vi "Kill All Notifiers.vi"() -> ()   [LabVIEW 2019]
uses:
  Globals and TypeDefs/Type Definitions.llb/McPherson Status.ctt
  Globals and TypeDefs/Type Definitions.llb/3 way Status.ctl
panel:
  in  "Spectrometer Pos":T2
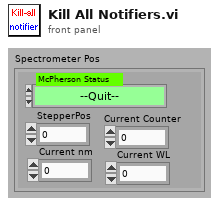
[diagram p1: front panel]
types:
  T1 = typedef "McPherson Status.ctt" = enum8{"--Quit--", "Error", "Initialization", "Standby", "Start Slew", "-Slew", "+Slew", "Slew Done", "Start Scan", "-Slew to Start", "+Slew to Start", "Scanning", "Scan Done", "Scan Pause", "Slew Pause", "Cancel", "Update Z0", "Sleep"}
  T2 = cluster{"StepperPos":i32, "Current nm":dbl, "Current Counter":dbl, "Current WL":dbl, "McPherson Status":T1}
  T3 = cluster{"Field [T]":dbl, "Status":cluster{bool, bool, "Ramp Status":u16, bool}}
  T4 = typedef "3 way Status.ctl" = u8
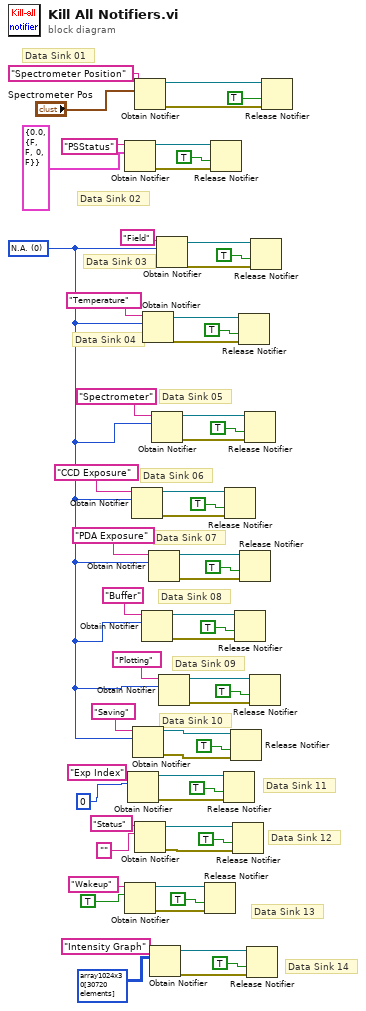
[diagram p0: block diagram]
diagram:
  w51 = T4 0 items=["N.A.", "OK", "Busy", "Done"] ("Saving")
  # "Data Sink 14"
  # "Data Sink 13"
  # "Data Sink 12"
  # "Data Sink 11"
  # "Data Sink 10"
  # "Data Sink 09"
  # "Data Sink 08"
  # "Data Sink 07"
  # "Data Sink 06"
  # "Data Sink 05"
  # "Data Sink 04"
  # "Data Sink 03"
  # "Data Sink 02"
  # "Data Sink 01"
  n1 = Obtain Notifier(name (unnamed)="PSStatus", notification data type=T3 {"Field [T]"=0.0, "Status"={FALSE, FALSE, "Ramp Status"=0, FALSE}} ("output cluster")) -> (notifier out=w37:refnum<notifier>, error out=w36:errorcluster)  [unwired: 2 in, 1 out]
  n2 = Obtain Notifier(name (unnamed)="Wakeup", notification data type=TRUE) -> (notifier out=w41:refnum<notifier>, error out=w39:errorcluster)  [unwired: 2 in, 1 out]
  n3 = Obtain Notifier(name (unnamed)="Exp Index", notification data type=u32 0 ("Exp Index")) -> (notifier out=w31:refnum<notifier>, error out=w30:errorcluster)  [unwired: 2 in, 1 out]
  n4 = Obtain Notifier(name (unnamed)="CCD Exposure", notification data type=w51) -> (notifier out=w19:refnum<notifier>, error out=w18:errorcluster)  [unwired: 2 in, 1 out]
  n5 = Obtain Notifier(name (unnamed)="Saving", notification data type=w51) -> (notifier out=w10:refnum<notifier>, error out=w9:errorcluster)  [unwired: 2 in, 1 out]
  n6 = Obtain Notifier(name (unnamed)="Spectrometer Position", notification data type="Spectrometer Pos") -> (notifier out=w45:refnum<notifier>, error out=w44:errorcluster)  [unwired: 2 in, 1 out]
  n7 = Obtain Notifier(name (unnamed)="Status", notification data type="" ("Status")) -> (notifier out=w7:refnum<notifier>, error out=w6:errorcluster)  [unwired: 2 in, 1 out]
  n8 = Obtain Notifier(name (unnamed)="Buffer", notification data type=w51) -> (notifier out=w16:refnum<notifier>, error out=w15:errorcluster)  [unwired: 2 in, 1 out]
  n9 = Obtain Notifier(name (unnamed)="Temperature", notification data type=w51) -> (notifier out=w25:refnum<notifier>, error out=w24:errorcluster)  [unwired: 2 in, 1 out]
  n10 = Obtain Notifier(name (unnamed)="PDA Exposure", notification data type=w51) -> (notifier out=w34:refnum<notifier>, error out=w33:errorcluster)  [unwired: 2 in, 1 out]
  n11 = Obtain Notifier(name (unnamed)="Intensity Graph", notification data type=i32[][] array1024x30[30720 elements] ("Intensity Graph")) -> (notifier out=w2:refnum<notifier>, error out=w1:errorcluster)  [unwired: 2 in, 1 out]
  n12 = Obtain Notifier(name (unnamed)="Spectrometer", notification data type=w51) -> (notifier out=w22:refnum<notifier>, error out=w21:errorcluster)  [unwired: 2 in, 1 out]
  n13 = Obtain Notifier(name (unnamed)="Field", notification data type=w51) -> (notifier out=w28:refnum<notifier>, error out=w27:errorcluster)  [unwired: 2 in, 1 out]
  n14 = Obtain Notifier(name (unnamed)="Plotting", notification data type=w51) -> (notifier out=w13:refnum<notifier>, error out=w12:errorcluster)  [unwired: 2 in, 1 out]
  n15 = Release Notifier(notifier=w41, force destroy? (F)=TRUE, error in (no error)=w39) -> ()  [unwired: 3 out]
  n16 = Release Notifier(notifier=w37, force destroy? (F)=TRUE, error in (no error)=w36) -> ()  [unwired: 3 out]
  n17 = Release Notifier(notifier=w31, force destroy? (F)=TRUE, error in (no error)=w30) -> ()  [unwired: 3 out]
  n18 = Release Notifier(notifier=w19, force destroy? (F)=TRUE, error in (no error)=w18) -> ()  [unwired: 3 out]
  n19 = Release Notifier(notifier=w10, force destroy? (F)=TRUE, error in (no error)=w9) -> ()  [unwired: 3 out]
  n20 = Release Notifier(notifier=w7, force destroy? (F)=TRUE, error in (no error)=w6) -> ()  [unwired: 3 out]
  n21 = Release Notifier(notifier=w16, force destroy? (F)=TRUE, error in (no error)=w15) -> ()  [unwired: 3 out]
  n22 = Release Notifier(notifier=w25, force destroy? (F)=TRUE, error in (no error)=w24) -> ()  [unwired: 3 out]
  n23 = Release Notifier(notifier=w34, force destroy? (F)=TRUE, error in (no error)=w33) -> ()  [unwired: 3 out]
  n24 = Release Notifier(notifier=w22, force destroy? (F)=TRUE, error in (no error)=w21) -> ()  [unwired: 3 out]
  n25 = Release Notifier(notifier=w2, force destroy? (F)=TRUE, error in (no error)=w1) -> ()  [unwired: 3 out]
  n26 = Release Notifier(notifier=w13, force destroy? (F)=TRUE, error in (no error)=w12) -> ()  [unwired: 3 out]
  n27 = Release Notifier(notifier=w28, force destroy? (F)=TRUE, error in (no error)=w27) -> ()  [unwired: 3 out]
  n28 = Release Notifier(notifier=w45, force destroy? (F)=TRUE, error in (no error)=w44) -> ()  [unwired: 3 out]
